vi "Channel Count.vi"(8 "error in (no error)":errorcluster, 11 "Thread Configuration in":refnum<class "Thread Configuration.lvclass">) -> (0 "error out":errorcluster, 2 "channel count":i32, 3 "Thread Configuration out":refnum<class "Thread Configuration.lvclass">)   [LabVIEW 2017, in "DSF Core.lvlib" / "Thread Configuration.lvclass"]
uses:
  Thread Configuration.lvclass
  Thread Configuration.lvclass/Thread Configuration.ctl
  Group/Group Configuration.lvclass
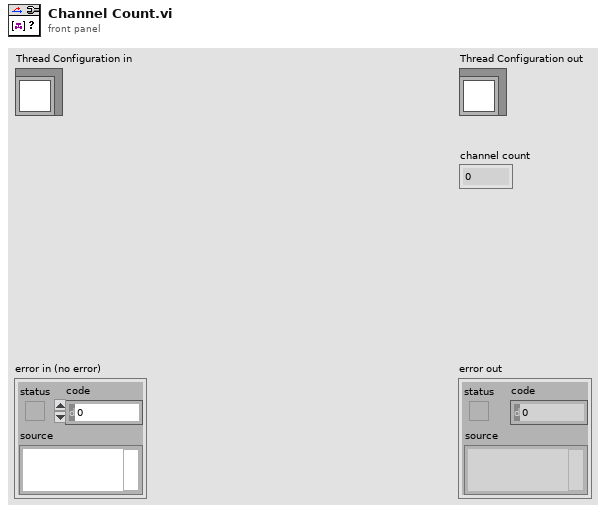
[diagram p1: front panel]
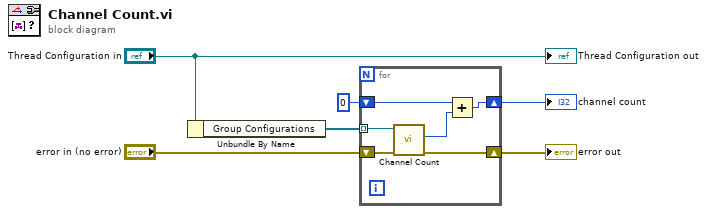
[diagram p0: block diagram]
diagram:
  n1 = Unbundle By Name("Thread Configuration in") -> ("Group Configurations"=w1:refnum<class "Group Configuration.lvclass">[])
  n2 = for {
    shift-right: [w11] -> w4
    shift-left: "error in (no error)" -> [w12]
    tunnel: w1 -> [w10] mode=indexing
    shift-right: [w7] -> w3
    shift-left: 0 ("channel count") -> [w9]
    n3 = call-dynamic "Channel Count.vi"("error in (no error)"=w12, "Group Configuration in"=w10) -> ("error out"=w11:errorcluster, "channel count"=w8:i32)  [unwired: 7 in, 1 out]
    n4 = Add(x=w9, y=w8) -> (x+y=w7:i32)
  }
  "error out" <- w4
  "channel count" <- w3
  "Thread Configuration out" <- "Thread Configuration in"
